vi "LoggingHeaders.vi"(8 "error in":errorcluster, 10 "Date and Time":string, 11 "refnum in":refnum<file>) -> (0 "error out":errorcluster, 3 "refnum out":refnum<file>)   [LabVIEW 2017]
uses:
  <vilib>/Rock Robotics/Network Tables/NT Read Number.vi
  <vilib>/Rock Robotics/Network Tables/NT Read String.vi
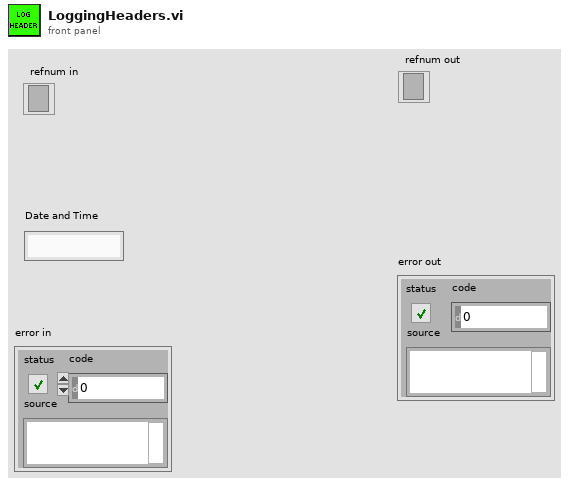
[diagram p1: front panel]
types:
  T1 = cluster{"Name":string, "Type":enum16{"Float", "Int", "Bool", "String"}}[]
  T2 = typedef "NetComm_MatchType.ctl" = enum32{"None", "Practice", "Qualification", "Elimination"}
  T3 = typedef "WPI_DriverStationPositionInfo.ctl" = enum16{"1", "2", "3"}
  T4 = typedef "WPI_DriverStationAllianceInfo.ctl" = enum16{"Red", "Blue", "Invalid"}
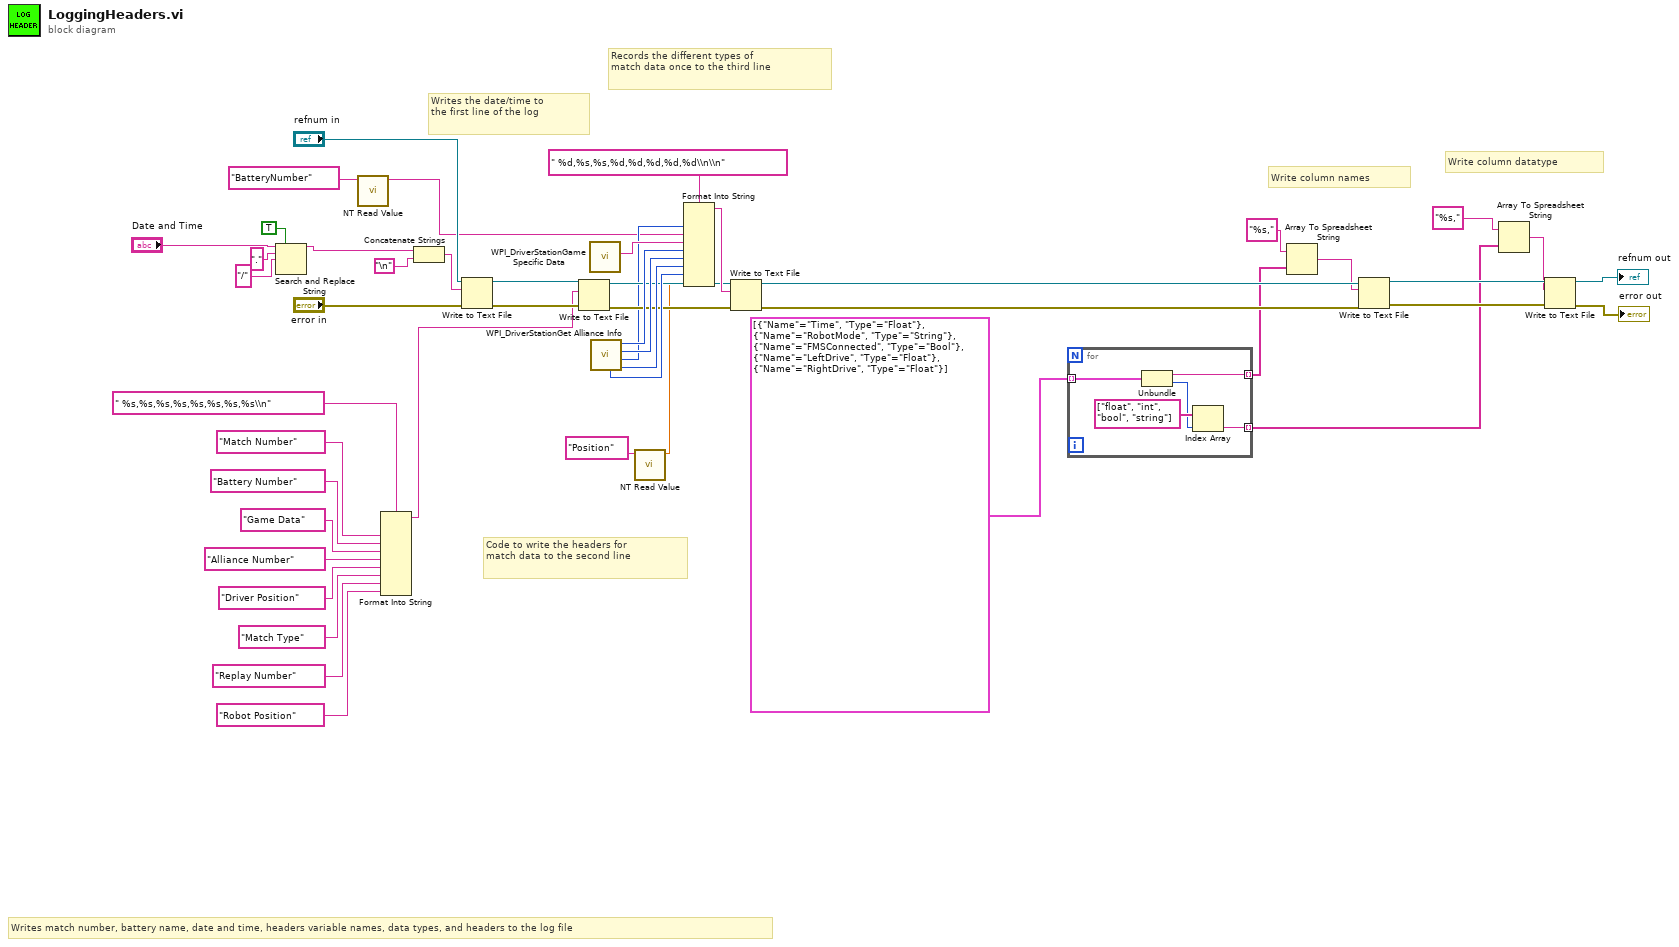
[diagram p0: block diagram]
diagram:
  # "Write column datatype"
  # "Write column names"
  # "Records the different types of \nmatch data once to the third line"
  # "Code to write the headers for \nmatch data to the second line"
  # "Writes the date/time to\nthe first line of the log"
  # "Writes match number, battery name, date and time, headers variable names, data types, and headers to the log file"
  n1 = Search and Replace String(replace all?=TRUE ("replace all? (F)"), input string="Date and Time", search string=".", replace string="/" ("search string")) -> (result string=w10:string)  [unwired: 4 in, 3 out]
  n2 = call-poly <vilib>:"NT Read Value.vi"("Name"="BatteryNumber") -> ("String"=w4:string)  [unwired: 9 in, 1 out]
  n3 = Format Into String(format string=" %s,%s,%s,%s,%s,%s,%s,%s\\n", "Match Number" ("input 2"), "Battery Number" ("input 2"), "Game Data" ("input 2"), "Alliance Number" ("input 2"), "Driver Position" ("input 2"), "Match Type" ("input 2"), "Replay Number" ("input 2"), "Robot Position" ("input 2")) -> (resulting string=w15:string)  [unwired: 2 in, 1 out]
  n4 = Concatenate Strings(w10, "\n") -> (w47:string)
  n5 = Write to Text File(file (use dialog)="refnum in", text=w47, error in="error in") -> (refnum out=w27:refnum<file>, error out=w26:errorcluster)  [unwired: 1 in, 1 out]
  n6 = Write to Text File(file (use dialog)=w27, text=w15, error in=w26) -> (refnum out=w24:refnum<file>, error out=w25:errorcluster)  [unwired: 1 in, 1 out]
  n7 = call <vilib>:"WPI_DriverStationGame Specific Data.vi"() -> ("Game Specific Data"=w32:string)  [unwired: 11 in]
  n8 = call <vilib>:"WPI_DriverStationGet Alliance Info.vi"() -> ("Match Type"=w29:T2, "Match Number"=w6:u16, "Position"=w30:T3, "Alliance"=w31:T4, "Replay Number"=w28:u16)  [unwired: 6 in, 1 out]
  n9 = call-poly <vilib>:"NT Read Value.vi"("Name"="Position") -> ("Numeric"=w7:dbl)  [unwired: 9 in, 1 out]
  n10 = Format Into String(format string=" %d,%s,%s,%d,%d,%d,%d,%d\\n\\n", w6, w4, w32, w31, w30, w29, w28, w7) -> (resulting string=w44:string)  [unwired: 2 in, 1 out]
  n11 = Write to Text File(file (use dialog)=w24, text=w44, error in=w25) -> (refnum out=w42:refnum<file>, error out=w41:errorcluster)  [unwired: 1 in, 1 out]
  n12 = for {
    tunnel: T1 [{"Name"="Time", "Type"=enum."Float"}, {"Name"="RobotMode", "Type"=enum."String"}, {"Name"="FMSConnected", "Type"=enum."Bool"}, {"Name"="LeftDrive", "Type"=enum."Float"}, {"Name"="RightDrive", "Type"=enum."Float"}] -> [w53] mode=indexing
    tunnel: [w50] -> w1 mode=indexing
    tunnel: [w49] -> w2 mode=indexing
    n13 = Unbundle(w53) -> ("Name"=w49:string, "Type"=w51:enum16{"Float", "Int", "Bool", "String"})
    n14 = Index Array(array=string[] ["float", "int", "bool", "string"] ("Name"), index=w51) -> (element=w50:string)
  }
  n15 = Array To Spreadsheet String(array=w2, 3:"%s," ("format string")) -> (spreadsheet string=w35:string)  [unwired: 1 in]
  n16 = Write to Text File(file (use dialog)=w42, text=w35, error in=w41) -> (refnum out=w39:refnum<file>, error out=w38:errorcluster)  [unwired: 1 in, 1 out]
  n17 = Array To Spreadsheet String(array=w1, 3:"%s," ("format string")) -> (spreadsheet string=w34:string)  [unwired: 1 in]
  n18 = Write to Text File(file (use dialog)=w39, text=w34, error in=w38) -> (refnum out=→"refnum out":refnum<file>, error out=→"error out":errorcluster)  [unwired: 1 in, 1 out]
